vi "GlobalStopPage1.vi"() -> ()   [LabVIEW 2013]
panel:
  out "stopPage1":bool
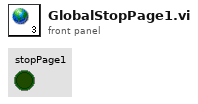
[diagram p1: front panel]
diagram:
